vi "Averaged DC-RMS.vi"   [LabVIEW 2020, in "NI_MAPro.lvlib"]
doc: "Calculates the DC and RMS values of an input waveform or array of waveforms. This VI is similar to the Basic Averaged DC-RMS VI, but this VI gives more precise control over the individual DC and RMS calculations."
uses:
  NI_MAPro.lvlib
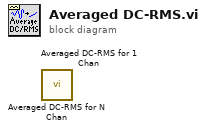
[diagram p0: block diagram]
diagram:
  n1 = call "Averaged DC-RMS for N Chan.vi"() -> ()  [unwired: 7 in, 5 out]
  n2 = call "Averaged DC-RMS for 1 Chan.vi"() -> ()  [unwired: 7 in, 5 out]
